vi "Parse Build-in Error Codes File Fields.vi"(8 "error in (no error)":errorcluster, 11 "errors file content in":string) -> (0 "error out":errorcluster, 1 "comment":string, 2 "family":T1, 3 "errors file content dup":string)   [LabVIEW 2017]
uses:
  Controls/NI Family.ctl
  <vilib>/regexp/Match Regular Expression.xnode
  Error File Management.lvlib
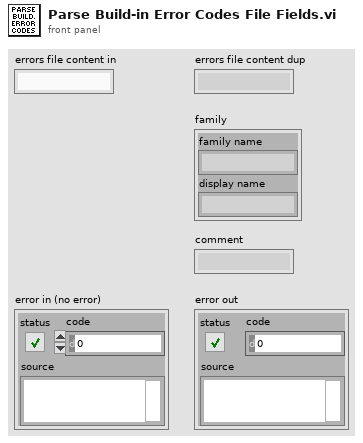
[diagram p1: front panel]
types:
  T1 = typedef "Error File Management.lvlib/NI Family.ctl" = cluster{"family name":string, "display name":string}
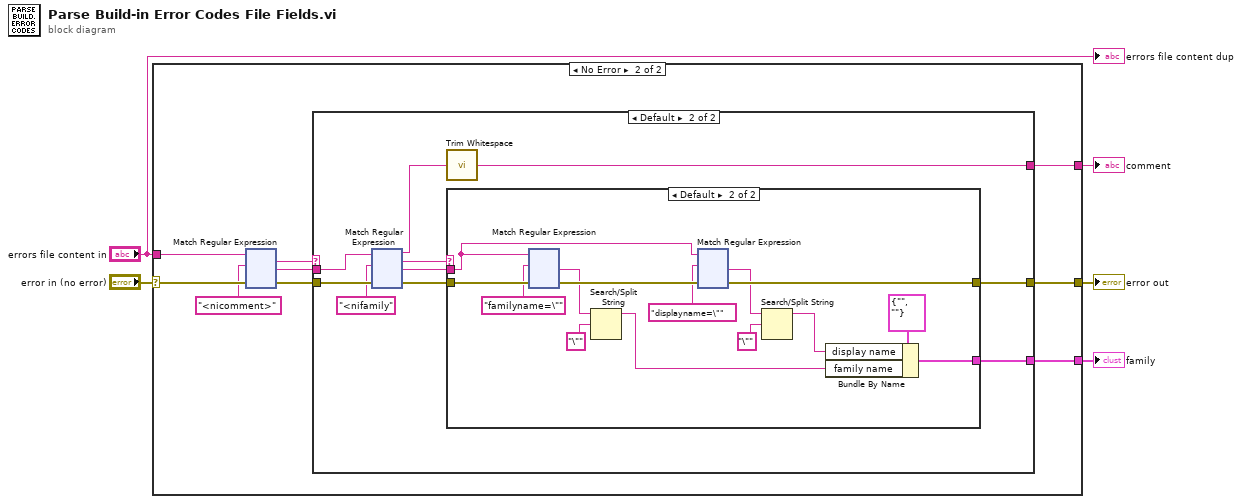
[diagram p0: block diagram]
diagram:
  n1 = case shown="No Error" "error in (no error)" {
    selector: "error in (no error)" -> [w6 w15]
    tunnel: [w6 w11] -> w4
    tunnel: [_ w10] -> w3
    tunnel: [_ w9] -> w2
    tunnel: "errors file content in" -> [_ w8]
    frame Error {
    }
    frame No Error {
      n2 = xnode "Match Regular Expression"("input string"=w8, "regular expression"="<nicomment>", "error in"=w15) -> ("whole match"=w13:string, "after match"=w7:string, "error out"=w12:errorcluster)  [unwired: 3 in, 2 out]
      n3 = case shown="Default" w13 {
        tunnel: [_ w23] -> w10
        tunnel: [_ w21] -> w9
        tunnel: w12 -> [w16 w26]
        tunnel: [w16 w19] -> w11
        tunnel: w7 -> [_ w18]
        frame "False" {
        }
        frame Default {
          n4 = xnode "Match Regular Expression"("input string"=w18, "regular expression"="<nifamily", "error in"=w26) -> ("before match"=w22:string, "whole match"=w24:string, "after match"=w17:string, "error out"=w20:errorcluster)  [unwired: 3 in, 1 out]
          n5 = call <vilib>:"Trim Whitespace.vi"("string"=w22) -> ("trimmed string"=w21:string)  [unwired: 1 in]
          n6 = case shown="Default" w24 {
            tunnel: [_ w34] -> w23
            tunnel: w20 -> [w27 w40]
            tunnel: [w27 w41] -> w19
            tunnel: w17 -> [_ w30]
            frame "False" {
            }
            frame Default {
              n7 = xnode "Match Regular Expression"("input string"=w30, "regular expression"="familyname=\"", "error in"=w40) -> ("after match"=w29:string, "error out"=w39:errorcluster)  [unwired: 3 in, 3 out]
              n8 = Search/Split String(string=w29, search string/char (-)="\"") -> (substring before match=w31:string)  [unwired: 1 in, 2 out]
              n9 = xnode "Match Regular Expression"("input string"=w30, "regular expression"="displayname=\"", "error in"=w39) -> ("after match"=w28:string, "error out"=w41:errorcluster)  [unwired: 3 in, 3 out]
              n10 = Search/Split String(string=w28, search string/char (-)="\"") -> (substring before match=w32:string)  [unwired: 1 in, 2 out]
              n11 = Bundle By Name(cluster=T1 {"family name"="", "display name"=""} ("family"), "display name"=w32, "family name"=w31) -> (w34:T1)
            }
          }
        }
      }
    }
  }
  "error out" <- w4
  "family" <- w3
  "comment" <- w2
  "errors file content dup" <- "errors file content in"
